vi "Request Data JSON.vi"(8 "error in (no error)":errorcluster, 11 "SetCurrentProgramScene in":refnum<class "SetCurrentProgramScene.lvclass">) -> (0 "error out":errorcluster, 2 "Request Data JSON":string, 3 "SetCurrentProgramScene out":refnum<class "SetCurrentProgramScene.lvclass">)   [LabVIEW 2022 SP3, in "obs-websocket-lv.lvlib" / "SetCurrentProgramScene.lvclass"]
uses:
  SetCurrentProgramScene.lvclass
  SetCurrentProgramScene.lvclass/SetCurrentProgramScene.ctl
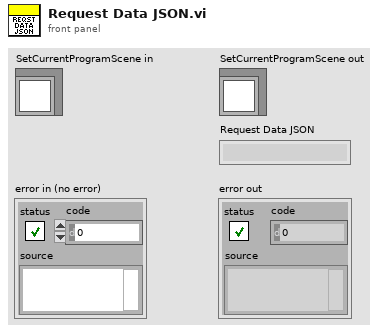
[diagram p1: front panel]
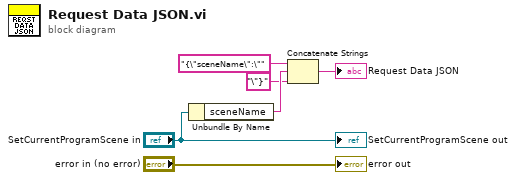
[diagram p0: block diagram]
diagram:
  n1 = Unbundle By Name("SetCurrentProgramScene in") -> ("sceneName"=w3:string)
  n2 = Concatenate Strings("{\"sceneName\":\"" ("string"), w3, "\"}" ("string")) -> (→"Request Data JSON":string)
  "error out" <- "error in (no error)"
  "SetCurrentProgramScene out" <- "SetCurrentProgramScene in"
